vi "point to dist.vi"(0 "Array 2":T9(array[cluster]), 1 "lock rcs value":cluster{"RCS 1":dbl, "RCS 2":dbl}, 2 "dist compensate":T3, 3 "lock RCS":bool, 5 "Cluster in":T8={"Direct program -1"={"Target 1"={"Boolean"=TRUE, "Speed"=100.0, "Range"=50.0, "Gain"=10.0}, "Target 2"={"Boolean"=FALSE, "Speed"=0.0, "Range"=0.0, "Gain"=0.0}, "Target 3"={"Boolean"=FALSE, "Speed"=0.0, "Range"=0.0, "Gain"=0.0}, "Target 4"={"Boolean"=FALSE, "Speed"=0.0, "Range"=0.0, "Gain"=0.0}}, "Direct program -2"={"Target 1"={"Boolean"=TRUE, "Speed"=100.0, "Range"=50.0, "Gain"=10.0}, "Target 2"={"Boolean"=FALSE, "Speed"=0.0, "Range"=0.0, "Gain"=0.0}, "Target 3"={"Boolean"=FALSE, "Speed"=0.0, "Range"=0.0, "Gain"=0.0}, "Target 4"={"Boolean"=FALSE, "Speed"=0.0, "Range"=0.0, "Gain"=0.0}}}, 9 "output cluster":T4, 11 "RCS":cluster{"Value":dbl, "Value":dbl}, 12 "DYNAMIC":T2(array[cluster]), 13 "DYNAMIC 2":T2(array[cluster])) -> (4 "1point":T7(array[cluster])=[[{"Vel"=0.0, "distance"=32.091545615629045, "angle"=30.256437163529274, "rad"=0.5280744484263598}, {"Vel"=0.0, "distance"=61.55057270245339, "angle"=48.93929886988103, "rad"=0.8541518988969639}, {"Vel"=0.0, "distance"=89.0740388665519, "angle"=40.72966957241671, "rad"=0.7108668372880226}, {"Vel"=0.0, "distance"=111.00188872266993, "angle"=31.573686861851996, "rad"=0.5510647927329934}, {"Vel"=0.0, "distance"=92.250607586075, "angle"=10.688712503953353, "rad"=0.18655322599307342}], [{"Vel"=0.0, "distance"=37.28981764503549, "angle"=23.333764643198865, "rad"=0.4072510199092601}, {"Vel"=0.0, "distance"=61.662336154252216, "angle"=54.80473394711968, "rad"=0.9565230530567463}, {"Vel"=0.0, "distance"=83.39019846480761, "angle"=38.19195784662725, "rad"=0.6665754122065289}, {"Vel"=0.0, "distance"=112.21265525777383, "angle"=28.30075576600638, "rad"=0.49394136891958124}, {"Vel"=0.0, "distance"=112.15762123012418, "angle"=9.742827579680815, "rad"=0.1700444197195404}]], 6 "Cluster  out":T8={"Direct program -1"={"Target 1"={"Boolean"=TRUE, "Speed"=100.0, "Range"=50.0, "Gain"=10.0}, "Target 2"={"Boolean"=FALSE, "Speed"=0.0, "Range"=0.0, "Gain"=0.0}, "Target 3"={"Boolean"=FALSE, "Speed"=0.0, "Range"=0.0, "Gain"=0.0}, "Target 4"={"Boolean"=FALSE, "Speed"=0.0, "Range"=0.0, "Gain"=0.0}}, "Direct program -2"={"Target 1"={"Boolean"=TRUE, "Speed"=100.0, "Range"=50.0, "Gain"=10.0}, "Target 2"={"Boolean"=FALSE, "Speed"=0.0, "Range"=0.0, "Gain"=0.0}, "Target 3"={"Boolean"=FALSE, "Speed"=0.0, "Range"=0.0, "Gain"=0.0}, "Target 4"={"Boolean"=FALSE, "Speed"=0.0, "Range"=0.0, "Gain"=0.0}}}, 10 "2 point":T7(array[cluster]), 14 "xy dynamic array":T1(array[cluster]), 15 "1to4":T6)   [LabVIEW 2015]
panel:
  out "Array":T5(array[cluster])
  in  "RCS":dbl
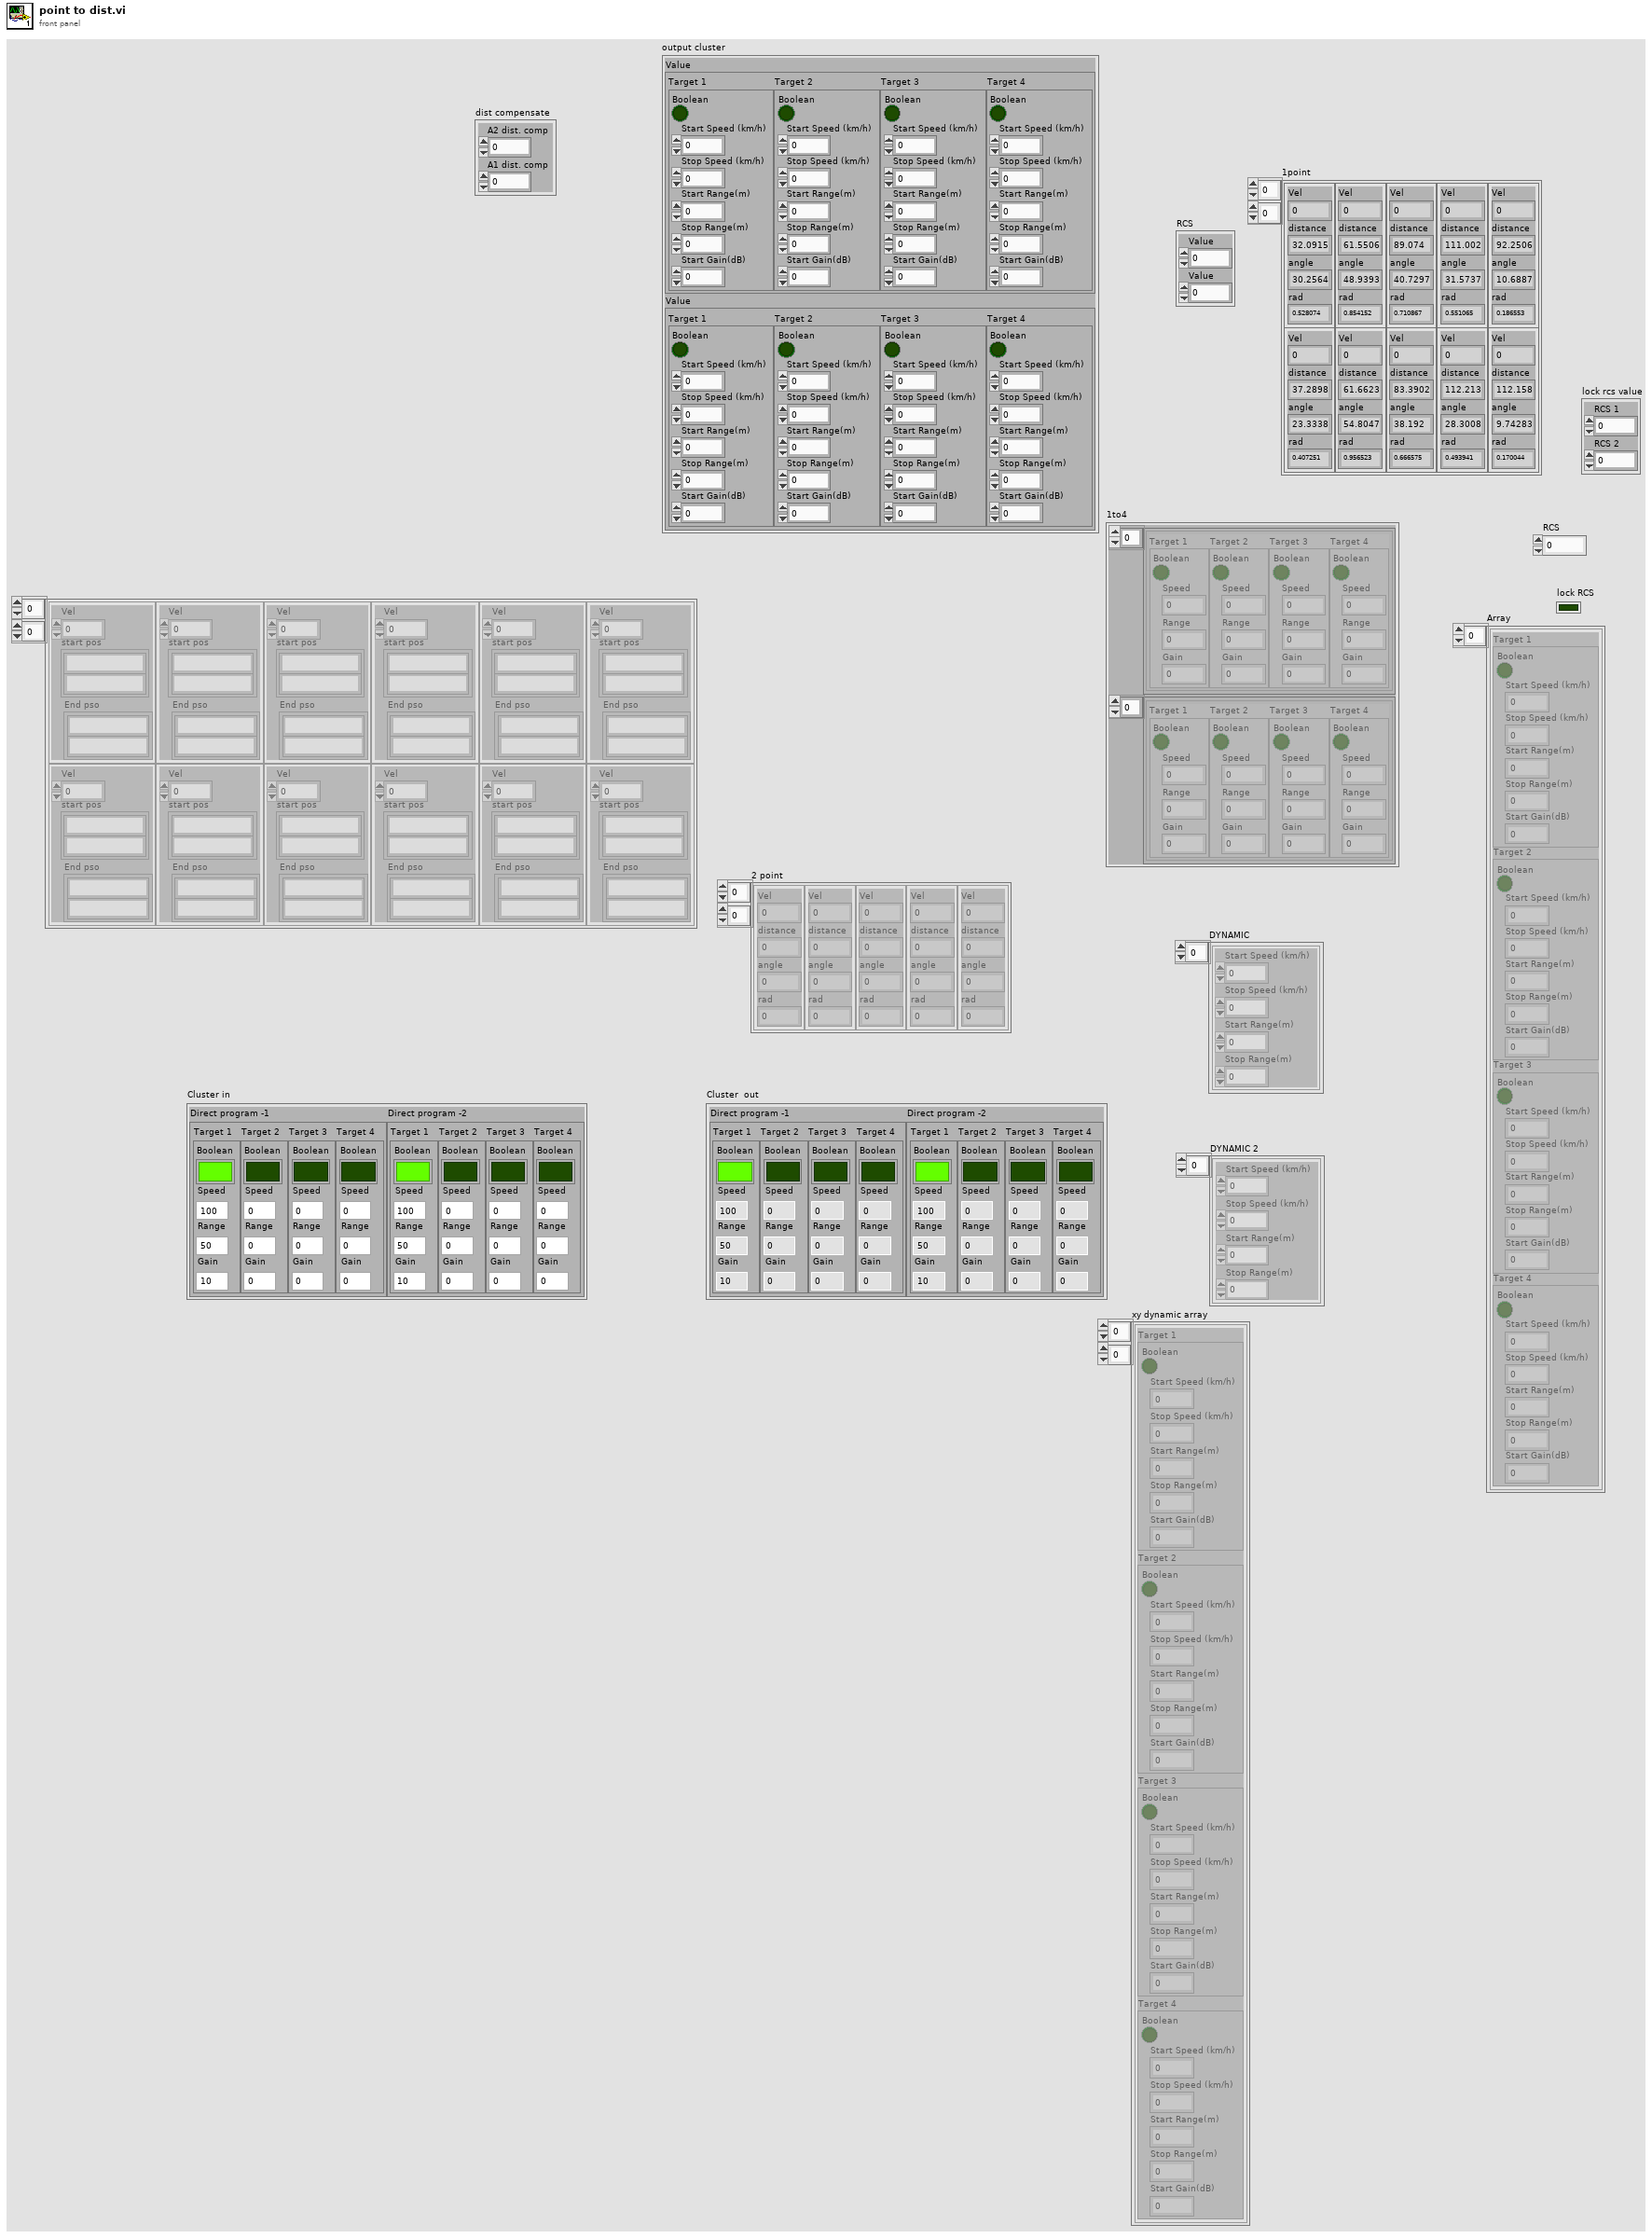
[diagram p1: front panel]
types:
  T1 = cluster{"Target 1":cluster{"Boolean":bool, "Start Speed (km/h)":dbl, "Stop Speed (km/h)":dbl, "Start Range(m)":dbl, "Stop Range(m)":dbl, "Start Gain(dB)":dbl}, "Target 2":cluster{"Boolean":bool, "Start Speed (km/h)":dbl, "Stop Speed (km/h)":dbl, "Start Range(m)":dbl, "Stop Range(m)":dbl, "Start Gain(dB)":dbl}, "Target 3":cluster{"Boolean":bool, "Start Speed (km/h)":dbl, "Stop Speed (km/h)":dbl, "Start Range(m)":dbl, "Stop Range(m)":dbl, "Start Gain(dB)":dbl}, "Target 4":cluster{"Boolean":bool, "Start Speed (km/h)":dbl, "Stop Speed (km/h)":dbl, "Start Range(m)":dbl, "Stop Range(m)":dbl, "Start Gain(dB)":dbl}}[][]
  T2 = cluster{"Start Speed (km/h)":dbl, "Stop Speed (km/h) ":dbl, "Start Range(m)":dbl, "Stop Range(m)":dbl}[]
  T3 = cluster{"A2 dist. comp":dbl, "A1 dist. comp":dbl}
  T4 = cluster{"Value":cluster{"Target 1":cluster{"Boolean":bool, "Start Speed (km/h)":dbl, "Stop Speed (km/h)":dbl, "Start Range(m)":dbl, "Stop Range(m)":dbl, "Start Gain(dB)":dbl}, "Target 2":cluster{"Boolean":bool, "Start Speed (km/h)":dbl, "Stop Speed (km/h)":dbl, "Start Range(m)":dbl, "Stop Range(m)":dbl, "Start Gain(dB)":dbl}, "Target 3":cluster{"Boolean":bool, "Start Speed (km/h)":dbl, "Stop Speed (km/h)":dbl, "Start Range(m)":dbl, "Stop Range(m)":dbl, "Start Gain(dB)":dbl}, "Target 4":cluster{"Boolean":bool, "Start Speed (km/h)":dbl, "Stop Speed (km/h)":dbl, "Start Range(m)":dbl, "Stop Range(m)":dbl, "Start Gain(dB)":dbl}}, "Value":cluster{"Target 1":cluster{"Boolean":bool, "Start Speed (km/h)":dbl, "Stop Speed (km/h)":dbl, "Start Range(m)":dbl, "Stop Range(m)":dbl, "Start Gain(dB)":dbl}, "Target 2":cluster{"Boolean":bool, "Start Speed (km/h)":dbl, "Stop Speed (km/h)":dbl, "Start Range(m)":dbl, "Stop Range(m)":dbl, "Start Gain(dB)":dbl}, "Target 3":cluster{"Boolean":bool, "Start Speed (km/h)":dbl, "Stop Speed (km/h)":dbl, "Start Range(m)":dbl, "Stop Range(m)":dbl, "Start Gain(dB)":dbl}, "Target 4":cluster{"Boolean":bool, "Start Speed (km/h)":dbl, "Stop Speed (km/h)":dbl, "Start Range(m)":dbl, "Stop Range(m)":dbl, "Start Gain(dB)":dbl}}}
  T5 = cluster{"Target 1":cluster{"Boolean":bool, "Start Speed (km/h)":dbl, "Stop Speed (km/h)":dbl, "Start Range(m)":dbl, "Stop Range(m)":dbl, "Start Gain(dB)":dbl}, "Target 2":cluster{"Boolean":bool, "Start Speed (km/h)":dbl, "Stop Speed (km/h)":dbl, "Start Range(m)":dbl, "Stop Range(m)":dbl, "Start Gain(dB)":dbl}, "Target 3":cluster{"Boolean":bool, "Start Speed (km/h)":dbl, "Stop Speed (km/h)":dbl, "Start Range(m)":dbl, "Stop Range(m)":dbl, "Start Gain(dB)":dbl}, "Target 4":cluster{"Boolean":bool, "Start Speed (km/h)":dbl, "Stop Speed (km/h)":dbl, "Start Range(m)":dbl, "Stop Range(m)":dbl, "Start Gain(dB)":dbl}}[]
  T6 = cluster{cluster{"Target 1":cluster{"Boolean":bool, "Speed":dbl, "Range":dbl, "Gain":dbl}, "Target 2":cluster{"Boolean":bool, "Speed":dbl, "Range":dbl, "Gain":dbl}, "Target 3":cluster{"Boolean":bool, "Speed":dbl, "Range":dbl, "Gain":dbl}, "Target 4":cluster{"Boolean":bool, "Speed":dbl, "Range":dbl, "Gain":dbl}}[], cluster{"Target 1":cluster{"Boolean":bool, "Speed":dbl, "Range":dbl, "Gain":dbl}, "Target 2":cluster{"Boolean":bool, "Speed":dbl, "Range":dbl, "Gain":dbl}, "Target 3":cluster{"Boolean":bool, "Speed":dbl, "Range":dbl, "Gain":dbl}, "Target 4":cluster{"Boolean":bool, "Speed":dbl, "Range":dbl, "Gain":dbl}}[]}
  T7 = cluster{"Vel":dbl, "distance":dbl, "angle":dbl, "rad":dbl}[][]
  T8 = cluster{"Direct program -1":cluster{"Target 1":cluster{"Boolean":bool, "Speed":dbl, "Range":dbl, "Gain":dbl}, "Target 2":cluster{"Boolean":bool, "Speed":dbl, "Range":dbl, "Gain":dbl}, "Target 3":cluster{"Boolean":bool, "Speed":dbl, "Range":dbl, "Gain":dbl}, "Target 4":cluster{"Boolean":bool, "Speed":dbl, "Range":dbl, "Gain":dbl}}, "Direct program -2":cluster{"Target 1":cluster{"Boolean":bool, "Speed":dbl, "Range":dbl, "Gain":dbl}, "Target 2":cluster{"Boolean":bool, "Speed":dbl, "Range":dbl, "Gain":dbl}, "Target 3":cluster{"Boolean":bool, "Speed":dbl, "Range":dbl, "Gain":dbl}, "Target 4":cluster{"Boolean":bool, "Speed":dbl, "Range":dbl, "Gain":dbl}}}
  T9 = cluster{"Vel":dbl, "start pos":cluster{string, string}, "End pso":cluster{string, string}}[][]
  T10 = cluster{"Target 1":cluster{"Boolean":bool, "Speed":dbl, "Range":dbl, "Gain":dbl}, "Target 2":cluster{"Boolean":bool, "Speed":dbl, "Range":dbl, "Gain":dbl}, "Target 3":cluster{"Boolean":bool, "Speed":dbl, "Range":dbl, "Gain":dbl}, "Target 4":cluster{"Boolean":bool, "Speed":dbl, "Range":dbl, "Gain":dbl}}
  T11 = cluster{"Vel":dbl, "start pos":cluster{string, string}, "End pso":cluster{string, string}}[]
  T12 = cluster{"Boolean":bool, "Speed":dbl, "Range":dbl, "Gain":dbl}
  T13 = cluster{"Target 1":cluster{"Boolean":bool, "Start Speed (km/h)":dbl, "Stop Speed (km/h)":dbl, "Start Range(m)":dbl, "Stop Range(m)":dbl, "Start Gain(dB)":dbl}, "Target 2":cluster{"Boolean":bool, "Start Speed (km/h)":dbl, "Stop Speed (km/h)":dbl, "Start Range(m)":dbl, "Stop Range(m)":dbl, "Start Gain(dB)":dbl}, "Target 3":cluster{"Boolean":bool, "Start Speed (km/h)":dbl, "Stop Speed (km/h)":dbl, "Start Range(m)":dbl, "Stop Range(m)":dbl, "Start Gain(dB)":dbl}, "Target 4":cluster{"Boolean":bool, "Start Speed (km/h)":dbl, "Stop Speed (km/h)":dbl, "Start Range(m)":dbl, "Stop Range(m)":dbl, "Start Gain(dB)":dbl}}
  T14 = cluster{cluster{"Target 1":cluster{"Boolean":bool, "Speed":dbl, "Range":dbl, "Gain":dbl}, "Target 2":cluster{"Boolean":bool, "Speed":dbl, "Range":dbl, "Gain":dbl}, "Target 3":cluster{"Boolean":bool, "Speed":dbl, "Range":dbl, "Gain":dbl}, "Target 4":cluster{"Boolean":bool, "Speed":dbl, "Range":dbl, "Gain":dbl}}, cluster{"Target 1":cluster{"Boolean":bool, "Speed":dbl, "Range":dbl, "Gain":dbl}, "Target 2":cluster{"Boolean":bool, "Speed":dbl, "Range":dbl, "Gain":dbl}, "Target 3":cluster{"Boolean":bool, "Speed":dbl, "Range":dbl, "Gain":dbl}, "Target 4":cluster{"Boolean":bool, "Speed":dbl, "Range":dbl, "Gain":dbl}}}
  T15 = cluster{"Boolean":bool, "Start Speed (km/h)":dbl, "Stop Speed (km/h)":dbl, "Start Range(m)":dbl, "Stop Range(m)":dbl, "Start Gain(dB)":dbl}
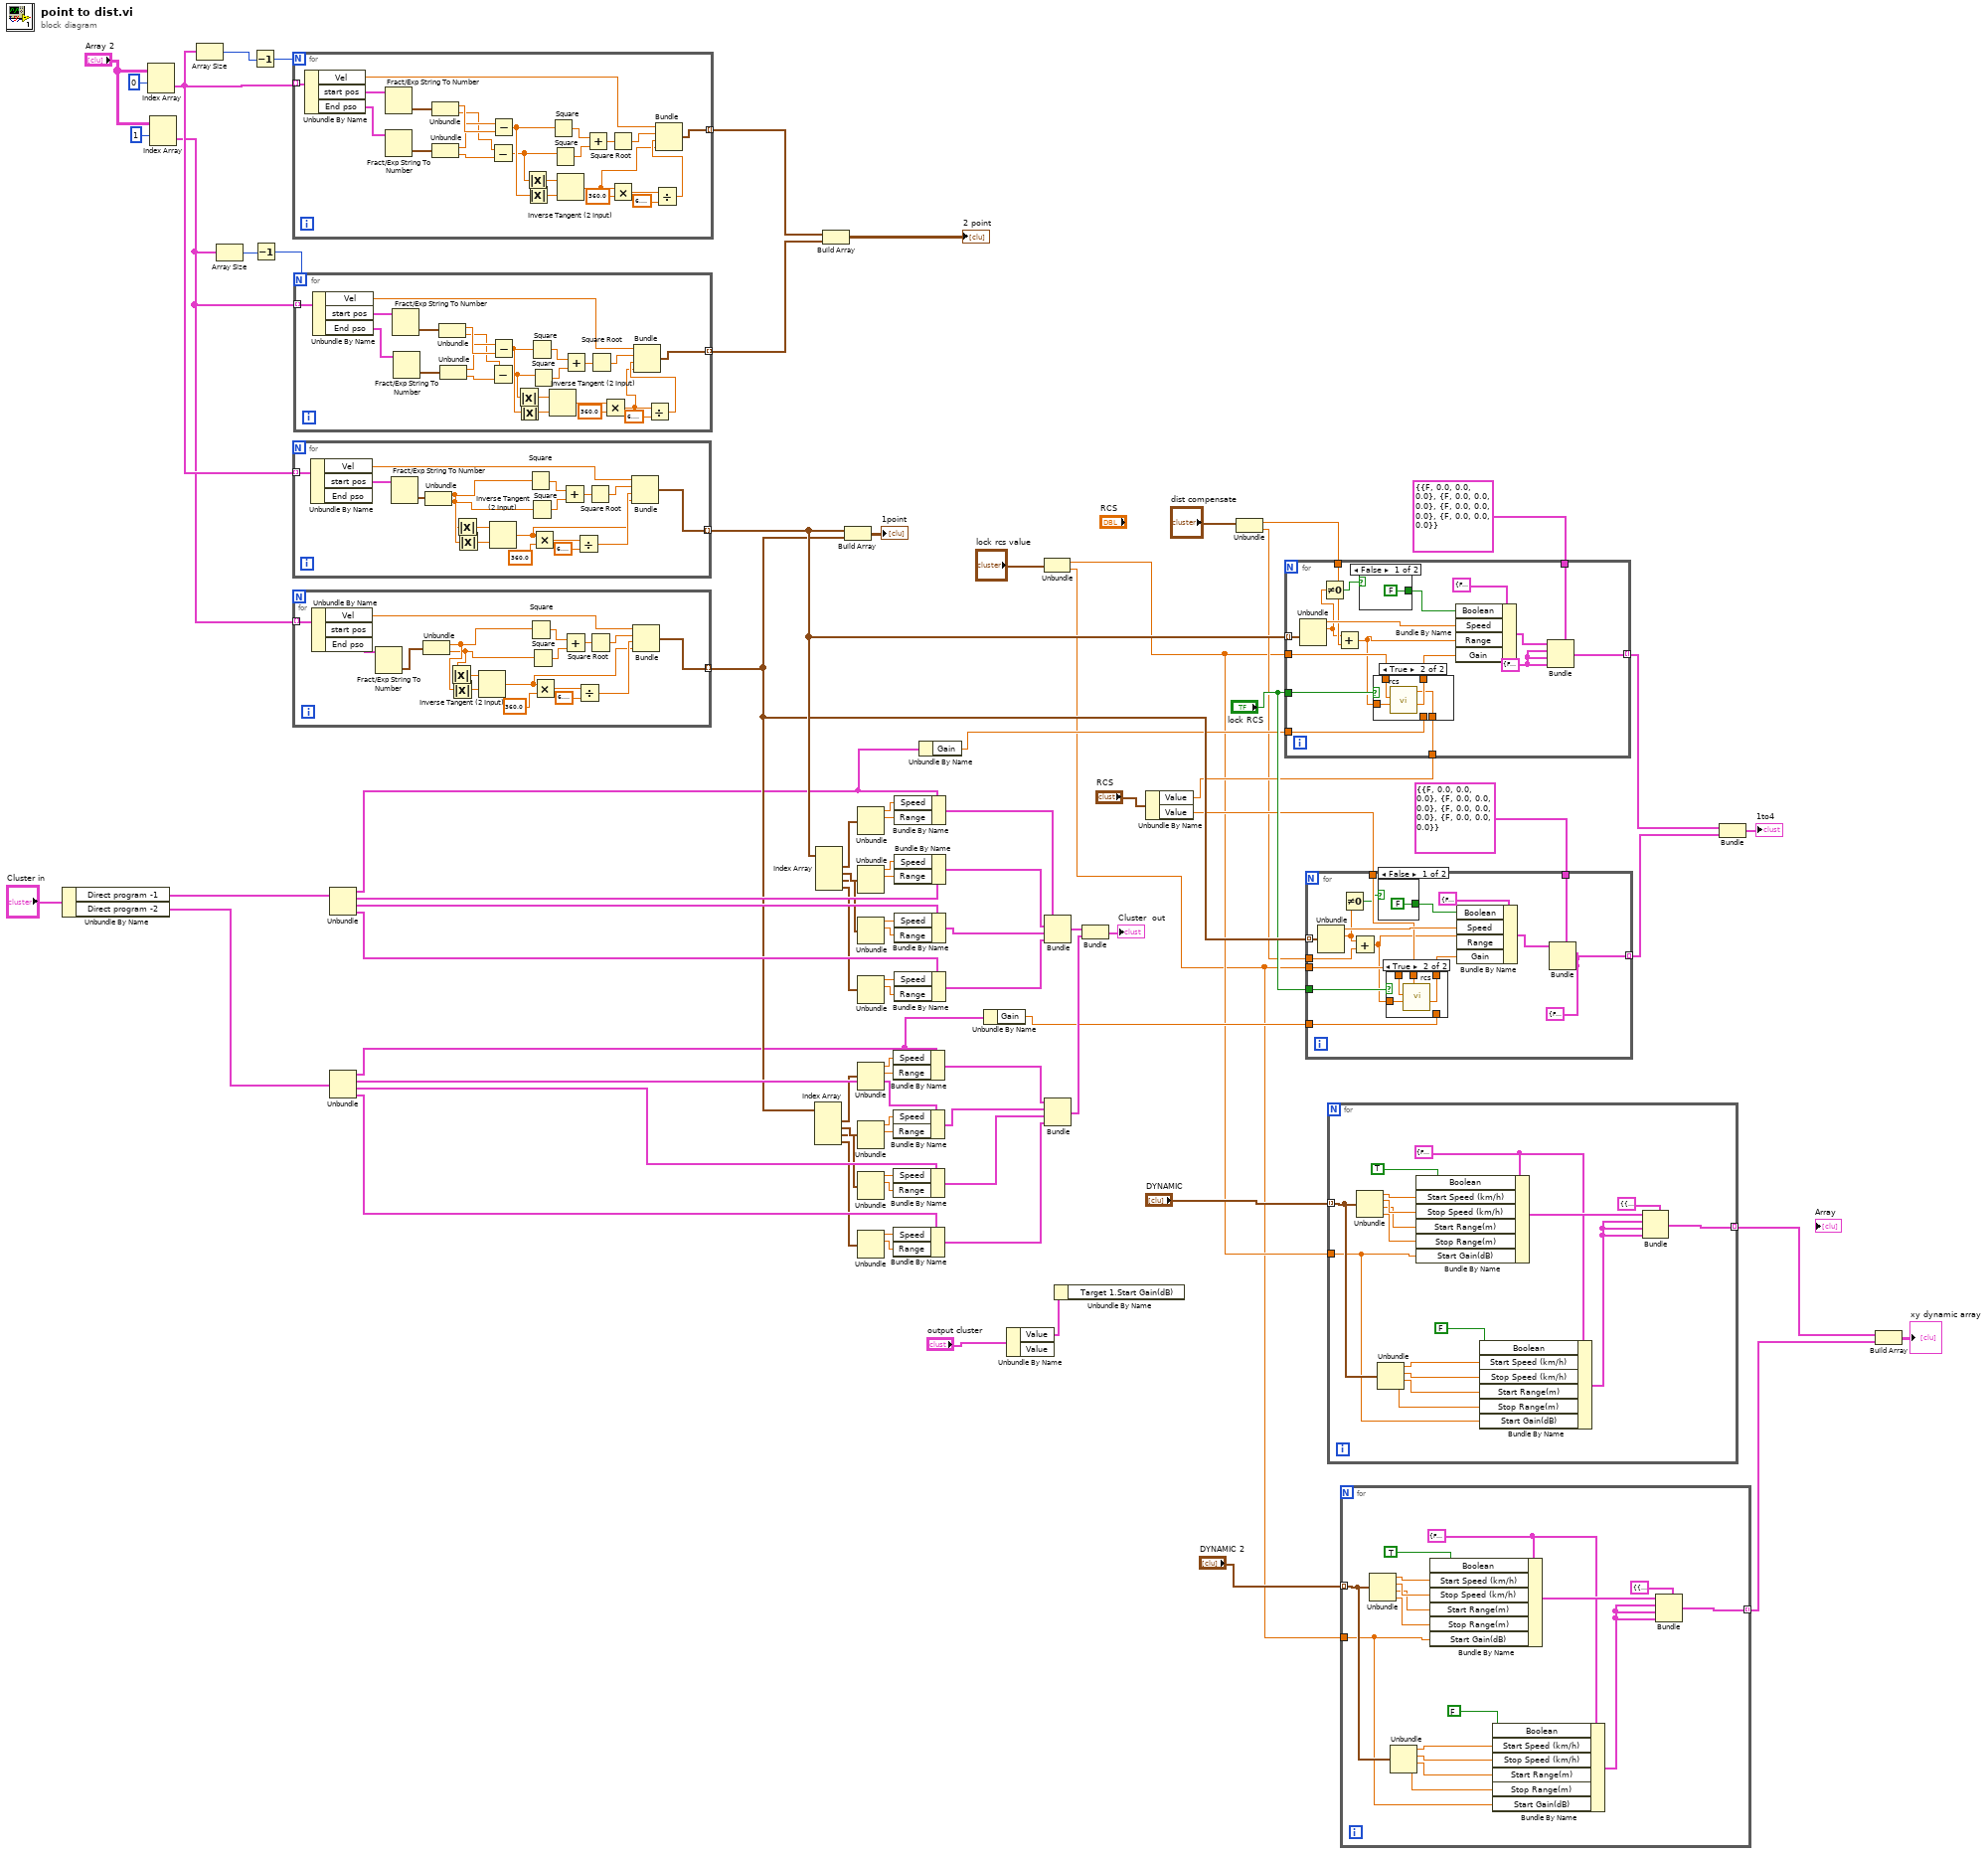
[diagram p0: block diagram]
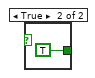
[diagram p2: hidden frame]
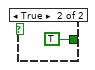
[diagram p4: hidden frame]
diagram:
  n1 = Unbundle By Name("Cluster in") -> ("Direct program -1"=w77:T10, "Direct program -2"=w63:T10)
  n2 = Index Array(array="Array 2", index (row)=0) -> (element=w36:T11)  [unwired: 1 in]
  n3 = Index Array(array="Array 2", index (row)=1) -> (element=w35:T11)  [unwired: 1 in]
  n4 = Array Size(array=w36) -> (size(s)=w81:i32)
  n5 = Array Size(array=w35) -> (size(s)=w80:i32)
  n6 = Decrement(x=w81) -> (x-1=w82:i32)
  n7 = Decrement(x=w80) -> (x-1=w79:i32)
  n8 = for {
    N: w82 -> [_]
    tunnel: w36 -> [w109] mode=indexing
    tunnel: [w90] -> w62 mode=indexing
    n9 = Unbundle By Name(w109) -> ("Vel"=w96:dbl, "start pos"=w108:cluster{string, string}, "End pso"=w107:cluster{string, string})
    n10 = Fract/Exp String To Number(string=w108) -> (number=w106:cluster{dbl, dbl})  [unwired: 3 in, 1 out]
    n11 = Fract/Exp String To Number(string=w107) -> (number=w105:cluster{dbl, dbl})  [unwired: 3 in, 1 out]
    n12 = Unbundle(w106) -> (w104:dbl, w102:dbl)
    n13 = Unbundle(w105) -> (w103:dbl, w101:dbl)
    n14 = Subtract(x=w102, y=w101) -> (x-y=w86:dbl)
    n15 = Subtract(x=w103, y=w104) -> (x-y=w87:dbl)
    n16 = Absolute Value(x=w86) -> (abs(x)=w89:dbl)
    n17 = Absolute Value(x=w87) -> (abs(x)=w88:dbl)
    n18 = Square(x=w87) -> (x^2=w100:dbl)
    n19 = Square(x=w86) -> (x^2=w99:dbl)
    n20 = Inverse Tangent (2 Input)(1:w88, 2:w89) -> (0:w91:dbl)
    n21 = Add(x=w100, y=w99) -> (x+y=w98:dbl)
    n22 = Square Root(x=w98) -> (sqrt(x)=w97:dbl)
    n23 = Multiply(x=w91, y=360.0) -> (x*y=w94:dbl)
    n24 = Divide(x=w94, y=6.283185307179586) -> (x/y=w92:dbl)
    n25 = Bundle("Vel"=w96, w97, w92, w91) -> (w90:cluster{"Vel":dbl, dbl, dbl, dbl})  [unwired: 1 in]
  }
  n26 = for {
    tunnel: w36 -> [w127] mode=indexing
    tunnel: [w119] -> w28 mode=indexing
    n27 = Unbundle By Name(w127) -> ("Vel"=w120:dbl, "start pos"=w126:cluster{string, string})  [unwired: 1 out]
    n28 = Fract/Exp String To Number(string=w126) -> (number=w125:cluster{dbl, dbl})  [unwired: 3 in, 1 out]
    n29 = Unbundle(w125) -> (w111:dbl, w110:dbl)
    n30 = Absolute Value(x=w110) -> (abs(x)=w113:dbl)
    n31 = Absolute Value(x=w111) -> (abs(x)=w112:dbl)
    n32 = Inverse Tangent (2 Input)(1:w112, 2:w113) -> (0:w114:dbl)
    n33 = Square(x=w111) -> (x^2=w124:dbl)
    n34 = Square(x=w110) -> (x^2=w123:dbl)
    n35 = Multiply(x=w114, y=360.0) -> (x*y=w117:dbl)
    n36 = Add(x=w124, y=w123) -> (x+y=w122:dbl)
    n37 = Divide(x=w117, y=6.283185307179586) -> (x/y=w115:dbl)
    n38 = Square Root(x=w122) -> (sqrt(x)=w121:dbl)
    n39 = Bundle("Vel"=w120, w121, w115, w114) -> (w119:cluster{"Vel":dbl, dbl, dbl, dbl})  [unwired: 1 in]
  }
  n40 = for {
    tunnel: w35 -> [w145] mode=indexing
    tunnel: [w138] -> w25 mode=indexing
    n41 = Unbundle By Name(w145) -> ("Vel"=w139:dbl, "start pos"=w144:cluster{string, string})  [unwired: 1 out]
    n42 = Fract/Exp String To Number(string=w144) -> (number=w128:cluster{dbl, dbl})  [unwired: 3 in, 1 out]
    n43 = Unbundle(w128) -> (w130:dbl, w129:dbl)
    n44 = Absolute Value(x=w129) -> (abs(x)=w132:dbl)
    n45 = Absolute Value(x=w130) -> (abs(x)=w131:dbl)
    n46 = Inverse Tangent (2 Input)(1:w131, 2:w132) -> (0:w133:dbl)
    n47 = Square(x=w130) -> (x^2=w143:dbl)
    n48 = Square(x=w129) -> (x^2=w142:dbl)
    n49 = Multiply(x=w133, y=360.0) -> (x*y=w136:dbl)
    n50 = Add(x=w143, y=w142) -> (x+y=w141:dbl)
    n51 = Divide(x=w136, y=6.283185307179586) -> (x/y=w134:dbl)
    n52 = Square Root(x=w141) -> (sqrt(x)=w140:dbl)
    n53 = Bundle("Vel"=w139, w140, w134, w133) -> (w138:cluster{"Vel":dbl, dbl, dbl, dbl})  [unwired: 1 in]
  }
  n54 = for {
    N: w79 -> [_]
    tunnel: w35 -> [w169] mode=indexing
    tunnel: [w150] -> w49 mode=indexing
    n55 = Unbundle By Name(w169) -> ("Vel"=w158:dbl, "start pos"=w168:cluster{string, string}, "End pso"=w167:cluster{string, string})
    n56 = Fract/Exp String To Number(string=w168) -> (number=w166:cluster{dbl, dbl})  [unwired: 3 in, 1 out]
    n57 = Fract/Exp String To Number(string=w167) -> (number=w165:cluster{dbl, dbl})  [unwired: 3 in, 1 out]
    n58 = Unbundle(w166) -> (w164:dbl, w162:dbl)
    n59 = Unbundle(w165) -> (w163:dbl, w161:dbl)
    n60 = Subtract(x=w162, y=w161) -> (x-y=w146:dbl)
    n61 = Subtract(x=w163, y=w164) -> (x-y=w147:dbl)
    n62 = Absolute Value(x=w146) -> (abs(x)=w149:dbl)
    n63 = Absolute Value(x=w147) -> (abs(x)=w148:dbl)
    n64 = Square(x=w147) -> (x^2=w153:dbl)
    n65 = Square(x=w146) -> (x^2=w154:dbl)
    n66 = Inverse Tangent (2 Input)(1:w148, 2:w149) -> (0:w155:dbl)
    n67 = Add(x=w153, y=w154) -> (x+y=w160:dbl)
    n68 = Square Root(x=w160) -> (sqrt(x)=w159:dbl)
    n69 = Multiply(x=w155, y=360.0) -> (x*y=w151:dbl)
    n70 = Divide(x=w151, y=6.283185307179586) -> (x/y=w152:dbl)
    n71 = Bundle("Vel"=w158, w159, w152, w151) -> (w150:cluster{"Vel":dbl, dbl, dbl, dbl})  [unwired: 1 in]
  }
  n72 = Unbundle(w77) -> ("Target 1"=w20:T12, "Target 2"=w76:T12, "Target 3"=w75:T12, "Target 4"=w74:T12)
  n73 = Unbundle(w63) -> ("Target 1"=w18:T12, "Target 2"=w68:T12, "Target 3"=w67:T12, "Target 4"=w66:T12)
  n74 = Index Array(array=w25) -> (element #1=w48:cluster{"Vel":dbl, dbl, dbl, dbl}, element #2=w47:cluster{"Vel":dbl, dbl, dbl, dbl}, element #3=w46:cluster{"Vel":dbl, dbl, dbl, dbl}, element #4=w45:cluster{"Vel":dbl, dbl, dbl, dbl})  [unwired: 4 in]
  n75 = Index Array(array=w28) -> (element #1=w61:cluster{"Vel":dbl, dbl, dbl, dbl}, element #2=w60:cluster{"Vel":dbl, dbl, dbl, dbl}, element #3=w59:cluster{"Vel":dbl, dbl, dbl, dbl}, element #4=w58:cluster{"Vel":dbl, dbl, dbl, dbl})  [unwired: 4 in]
  n76 = Build Array(w62, w49) -> (→"2 point":cluster{"Vel":dbl, dbl, dbl, dbl}[][])
  n77 = Build Array(w28, w25) -> (→"1point":cluster{"Vel":dbl, dbl, dbl, dbl}[][])
  n78 = Unbundle(w48) -> ("Vel"=w44:dbl, w37:dbl)  [unwired: 2 out]
  n79 = Unbundle(w47) -> ("Vel"=w43:dbl, w38:dbl)  [unwired: 2 out]
  n80 = Unbundle(w46) -> ("Vel"=w42:dbl, w39:dbl)  [unwired: 2 out]
  n81 = Unbundle(w45) -> ("Vel"=w41:dbl, w40:dbl)  [unwired: 2 out]
  n82 = Unbundle(w61) -> ("Vel"=w57:dbl, w53:dbl)  [unwired: 2 out]
  n83 = Unbundle(w60) -> ("Vel"=w56:dbl, w52:dbl)  [unwired: 2 out]
  n84 = Unbundle(w59) -> ("Vel"=w55:dbl, w51:dbl)  [unwired: 2 out]
  n85 = Unbundle(w58) -> ("Vel"=w54:dbl, w50:dbl)  [unwired: 2 out]
  n86 = Bundle By Name(cluster=w18, "Speed"=w44, "Range"=w37) -> (w72:T12)
  n87 = Bundle By Name(cluster=w68, "Speed"=w43, "Range"=w38) -> (w71:T12)
  n88 = Bundle By Name(cluster=w67, "Speed"=w42, "Range"=w39) -> (w70:T12)
  n89 = Bundle By Name(cluster=w66, "Speed"=w41, "Range"=w40) -> (w69:T12)
  n90 = Bundle By Name(cluster=w20, "Speed"=w57, "Range"=w53) -> (w29:T12)
  n91 = Bundle By Name(cluster=w76, "Speed"=w56, "Range"=w52) -> (w32:T12)
  n92 = Bundle By Name(cluster=w75, "Speed"=w55, "Range"=w51) -> (w31:T12)
  n93 = Bundle By Name(cluster=w74, "Speed"=w54, "Range"=w50) -> (w30:T12)
  n94 = Unbundle By Name(w20) -> ("Gain"=w19:dbl)
  n95 = Unbundle By Name(w18) -> ("Gain"=w17:dbl)
  n96 = Unbundle By Name("output cluster") -> ("Value"=w14:T13)  [unwired: 1 out]
  n97 = Unbundle("lock rcs value") -> ("RCS 1"=w6:dbl, "RCS 2"=w4:dbl)
  n98 = Bundle("Target 1"=w29, "Target 2"=w32, "Target 3"=w31, "Target 4"=w30) -> (w73:T10)  [unwired: 1 in]
  n99 = Bundle("Target 1"=w72, "Target 2"=w71, "Target 3"=w70, "Target 4"=w69) -> (w65:T10)  [unwired: 1 in]
  n100 = Unbundle By Name(w14) -> ()  [unwired: 1 out]
  n101 = Bundle(w73, w65) -> (→"Cluster  out":T14)  [unwired: 1 in]
  n102 = Unbundle By Name("RCS") -> ("Value"=w12:dbl, "Value"=w11:dbl)
  n103 = Unbundle("dist compensate") -> ("A2 dist. comp"=w8:dbl, "A1 dist. comp"=w7:dbl)
  n104 = for {
    tunnel: w28 -> [w186] mode=indexing
    tunnel: T10 {"Target 1"={"Boolean"=FALSE, "Speed"=0.0, "Range"=0.0, "Gain"=0.0}, "Target 2"={"Boolean"=FALSE, "Speed"=0.0, "Range"=0.0, "Gain"=0.0}, "Target 3"={"Boolean"=FALSE, "Speed"=0.0, "Range"=0.0, "Gain"=0.0}, "Target 4"={"Boolean"=FALSE, "Speed"=0.0, "Range"=0.0, "Gain"=0.0}} ("Direct program -1") -> [w183]
    tunnel: [w179] -> w24 mode=indexing
    tunnel: w6 -> [w177]
    tunnel: "lock RCS" -> [w176]
    tunnel: w19 -> [w175]
    tunnel: w12 -> [w174]
    tunnel: w8 -> [w172]
    w184 = T12 {"Boolean"=FALSE, "Speed"=0.0, "Range"=0.0, "Gain"=0.0} ("Target 1")
    n105 = Unbundle(w186) -> ("Vel"=w185:dbl, w170:dbl)  [unwired: 2 out]
    n106 = Not Equal To 0?(x=w170) -> (x != 0?=w171:bool)
    n107 = Add(x=w170, y=w172) -> (x+y=w173:dbl)
    n108 = case shown="False" w171 {
      tunnel: [FALSE ("Boolean") TRUE ("Boolean")] -> w181
      frame False {
      }
      frame True {
      }
    }
    n109 = case shown="True" w176 {
      tunnel: [w189 w193] -> w178
      tunnel: w177 -> [_ w192]
      tunnel: w173 -> [_ w191]
      tunnel: w175 -> [w189 _]
      tunnel: w174 -> [_ w190]
      frame False {
      }
      frame True {
        n110 = call "rcs.vi"("RCS REF"=w190, "range"=w191, "rcs"=w192) -> ("gain"=w193:dbl)  [unwired: 7 in, 1 out]
      }
    }
    n111 = Bundle By Name(cluster=T12 {"Boolean"=FALSE, "Speed"=0.0, "Range"=0.0, "Gain"=0.0} ("Target 1"), "Boolean"=w181, "Speed"=w185, "Range"=w173, "Gain"=w178) -> (w180:T12)
    n112 = Bundle(cluster=w183, "Target 1"=w180, "Target 2"=w184, "Target 3"=w184, "Target 4"=w184) -> (w179:T10)
  }
  n113 = for {
    tunnel: w25 -> [w210] mode=indexing
    tunnel: T10 {"Target 1"={"Boolean"=FALSE, "Speed"=0.0, "Range"=0.0, "Gain"=0.0}, "Target 2"={"Boolean"=FALSE, "Speed"=0.0, "Range"=0.0, "Gain"=0.0}, "Target 3"={"Boolean"=FALSE, "Speed"=0.0, "Range"=0.0, "Gain"=0.0}, "Target 4"={"Boolean"=FALSE, "Speed"=0.0, "Range"=0.0, "Gain"=0.0}} ("Direct program -1") -> [w207]
    tunnel: [w203] -> w23 mode=indexing
    tunnel: w4 -> [w202]
    tunnel: "lock RCS" -> [w200]
    tunnel: w17 -> [w199]
    tunnel: w11 -> [w198]
    tunnel: w7 -> [w196]
    w208 = T12 {"Boolean"=FALSE, "Speed"=0.0, "Range"=0.0, "Gain"=0.0} ("Target 1")
    n114 = Unbundle(w210) -> ("Vel"=w209:dbl, w194:dbl)  [unwired: 2 out]
    n115 = Not Equal To 0?(x=w194) -> (x != 0?=w195:bool)
    n116 = Add(x=w194, y=w196) -> (x+y=w197:dbl)
    n117 = case shown="False" w195 {
      tunnel: [FALSE ("Boolean") TRUE ("Boolean")] -> w205
      frame False {
      }
      frame True {
      }
    }
    n118 = case shown="True" w200 {
      tunnel: [w213 w217] -> w201
      tunnel: w202 -> [_ w216]
      tunnel: w197 -> [_ w215]
      tunnel: w199 -> [w213 _]
      tunnel: w198 -> [_ w214]
      frame False {
      }
      frame True {
        n119 = call "rcs.vi"("RCS REF"=w214, "range"=w215, "rcs"=w216) -> ("gain"=w217:dbl)  [unwired: 7 in, 1 out]
      }
    }
    n120 = Bundle By Name(cluster=T12 {"Boolean"=FALSE, "Speed"=0.0, "Range"=0.0, "Gain"=0.0} ("Target 1"), "Boolean"=w205, "Speed"=w209, "Range"=w197, "Gain"=w201) -> (w204:T12)
    n121 = Bundle(cluster=w207, "Target 1"=w204, "Target 2"=w208, "Target 3"=w208, "Target 4"=w208) -> (w203:T10)
  }
  n122 = for {
    tunnel: "DYNAMIC" -> [w224] mode=indexing
    tunnel: [w231] -> w3 mode=indexing
    tunnel: w6 -> [w219]
    w226 = T15 {"Boolean"=FALSE, "Start Speed (km/h)"=0.0, "Stop Speed (km/h)"=0.0, "Start Range(m)"=0.0, "Stop Range(m)"=0.0, "Start Gain(dB)"=0.0} ("Target 4")
    n123 = Unbundle(w224) -> ("Start Speed (km/h)"=w230:dbl, "Stop Speed (km/h)"=w229:dbl, "Start Range(m)"=w228:dbl, "Stop Range(m)"=w227:dbl)
    n124 = Unbundle(w224) -> ("Start Speed (km/h)"=w223:dbl, "Stop Speed (km/h)"=w222:dbl, "Start Range(m)"=w221:dbl, "Stop Range(m)"=w220:dbl)
    n125 = Bundle By Name(cluster=w226, "Boolean"=TRUE, "Start Speed (km/h)"=w230, "Stop Speed (km/h)"=w229, "Start Range(m)"=w228, "Stop Range(m)"=w227, "Start Gain(dB)"=w219) -> (w232:T15)
    n126 = Bundle By Name(cluster=w226, "Boolean"=FALSE, "Start Speed (km/h)"=w223, "Stop Speed (km/h)"=w222, "Start Range(m)"=w221, "Stop Range(m)"=w220, "Start Gain(dB)"=w219) -> (w218:T15)
    n127 = Bundle(cluster=T13 {"Target 1"={"Boolean"=FALSE, "Start Speed (km/h)"=0.0, "Stop Speed (km/h)"=0.0, "Start Range(m)"=0.0, "Stop Range(m)"=0.0, "Start Gain(dB)"=0.0}, "Target 2"={"Boolean"=FALSE, "Start Speed (km/h)"=0.0, "Stop Speed (km/h)"=0.0, "Start Range(m)"=0.0, "Stop Range(m)"=0.0, "Start Gain(dB)"=0.0}, "Target 3"={"Boolean"=FALSE, "Start Speed (km/h)"=0.0, "Stop Speed (km/h)"=0.0, "Start Range(m)"=0.0, "Stop Range(m)"=0.0, "Start Gain(dB)"=0.0}, "Target 4"={"Boolean"=FALSE, "Start Speed (km/h)"=0.0, "Stop Speed (km/h)"=0.0, "Start Range(m)"=0.0, "Stop Range(m)"=0.0, "Start Gain(dB)"=0.0}} ("Dynamic"), "Target 1"=w232, "Target 2"=w218, "Target 3"=w218, "Target 4"=w218) -> (w231:T13)
  }
  n128 = for {
    tunnel: "DYNAMIC 2" -> [w241] mode=indexing
    tunnel: [w248] -> w2 mode=indexing
    tunnel: w4 -> [w236]
    w243 = T15 {"Boolean"=FALSE, "Start Speed (km/h)"=0.0, "Stop Speed (km/h)"=0.0, "Start Range(m)"=0.0, "Stop Range(m)"=0.0, "Start Gain(dB)"=0.0} ("Target 4")
    n129 = Unbundle(w241) -> ("Start Speed (km/h)"=w247:dbl, "Stop Speed (km/h)"=w246:dbl, "Start Range(m)"=w245:dbl, "Stop Range(m)"=w244:dbl)
    n130 = Unbundle(w241) -> ("Start Speed (km/h)"=w240:dbl, "Stop Speed (km/h)"=w239:dbl, "Start Range(m)"=w238:dbl, "Stop Range(m)"=w237:dbl)
    n131 = Bundle By Name(cluster=w243, "Boolean"=TRUE, "Start Speed (km/h)"=w247, "Stop Speed (km/h)"=w246, "Start Range(m)"=w245, "Stop Range(m)"=w244, "Start Gain(dB)"=w236) -> (w249:T15)
    n132 = Bundle By Name(cluster=w243, "Boolean"=FALSE, "Start Speed (km/h)"=w240, "Stop Speed (km/h)"=w239, "Start Range(m)"=w238, "Stop Range(m)"=w237, "Start Gain(dB)"=w236) -> (w235:T15)
    n133 = Bundle(cluster=T13 {"Target 1"={"Boolean"=FALSE, "Start Speed (km/h)"=0.0, "Stop Speed (km/h)"=0.0, "Start Range(m)"=0.0, "Stop Range(m)"=0.0, "Start Gain(dB)"=0.0}, "Target 2"={"Boolean"=FALSE, "Start Speed (km/h)"=0.0, "Stop Speed (km/h)"=0.0, "Start Range(m)"=0.0, "Stop Range(m)"=0.0, "Start Gain(dB)"=0.0}, "Target 3"={"Boolean"=FALSE, "Start Speed (km/h)"=0.0, "Stop Speed (km/h)"=0.0, "Start Range(m)"=0.0, "Stop Range(m)"=0.0, "Start Gain(dB)"=0.0}, "Target 4"={"Boolean"=FALSE, "Start Speed (km/h)"=0.0, "Stop Speed (km/h)"=0.0, "Start Range(m)"=0.0, "Stop Range(m)"=0.0, "Start Gain(dB)"=0.0}} ("Dynamic"), "Target 1"=w249, "Target 2"=w235, "Target 3"=w235, "Target 4"=w235) -> (w248:T13)
  }
  n134 = Bundle(w24, w23) -> (→"1to4":T6)  [unwired: 1 in]
  n135 = Build Array(w3, w2) -> (→"xy dynamic array":T1)
